vi "[GV]_Lidar 오브젝트화 된 배열.vi"() -> ()   [LabVIEW 2016, in "Lidar Variables.lvlib"]
uses:
  Lidar Variables.lvlib
panel:
  in  "오브젝트화된 배열(x,y)":dbl[][](array[numeric])
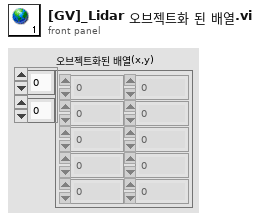
[diagram p1: front panel]
diagram:
